vi "Copy Buffer Example.vi"() -> ()   [LabVIEW 2012]
uses:
  User Controls/Array Dimensions.ctl
  User Controls/Copy Parameters.ctl
  User Controls/Offset.ctl
  Non-User VIs/Allocate Memory/AllocateMemory_u16.vi
  Non-User VIs/Write Memory/WriteMemory_u16.vi
  Non-User VIs/Read Memory/ReadMemory 16u .vi
  Non-User VIs/Error Checking/View Error Log Mode Functional Global.vi
  OpenCLV x64.lvlib
panel:
  out "Data Out":u16[][][](array[numeric])
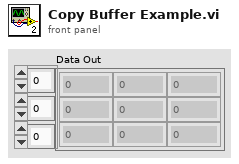
[diagram p1: front panel]
types:
  T1 = typedef "Copy Parameters.ctl" = cluster{"Source Offset":T2, "Destination Offset":T2, "Dimensions":T3}
  T2 = typedef "Offset.ctl" = cluster{"X":u64, "Y":u64, "Z":u64}
  T3 = typedef "Array Dimensions.ctl" = cluster{"Depth":u64, "Height":u64, "Width":u64}
  T4 = typedef "OpenCLV x64.lvlib/Device ID.ctl" = u64
  T5 = typedef "OpenCLV x64.lvlib/Memory Object.ctl" = cluster{"Device ID":T4, "Memeroy ID":T6, "Dimension":T3, "Memory Type":T7}
  T6 = typedef "OpenCLV x64.lvlib/Memory ID.ctl" = u64
  T7 = typedef "OpenCLV x64.lvlib/Memory Type.ctl" = enum16{"32f", "u8", "i8", "u16", "i16", "u32", "i32", "64f"}
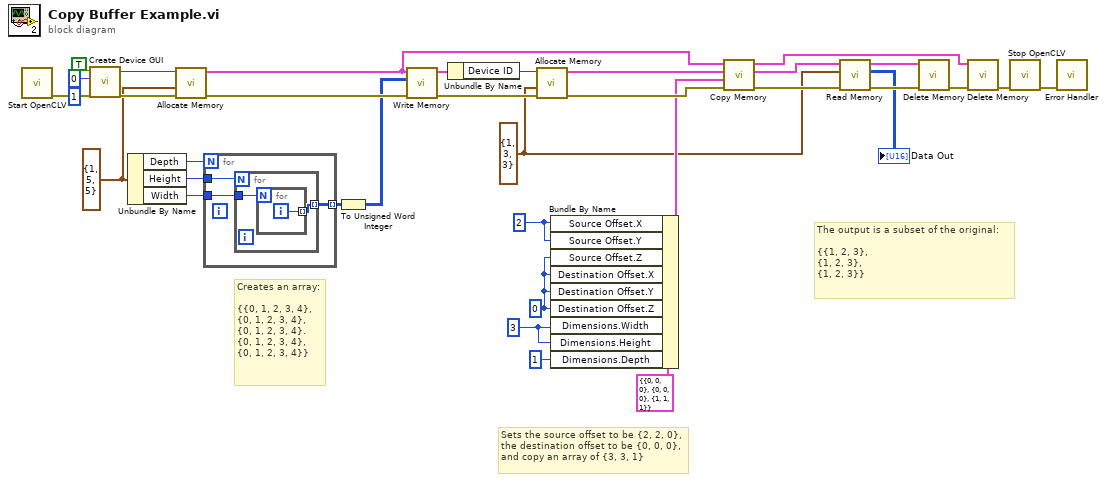
[diagram p0: block diagram]
diagram:
  w14 = u64 3 ("Dimensions.Width")
  w4 = u64 0 ("Destination Offset.Z")
  w3 = u64 2 ("Source Offset.X")
  w10 = T3 {"Depth"=1, "Height"=3, "Width"=3} ("Dimension")
  w29 = T3 {"Depth"=1, "Height"=5, "Width"=5} ("Dimension")
  # "The output is a subset of the original:\n\n{{1, 2, 3},\n{1, 2, 3},\n{1, 2, 3}}"
  # "Sets the source offset to be {2, 2, 0},\nthe destination offset to be {0, 0, 0},\nand copy an array of {3, 3, 1}"
  # "Creates an array:\n\n{{0, 1, 2, 3, 4},\n{0, 1, 2, 3, 4},\n{0, 1, 2, 3, 4}.\n{0, 1, 2, 3, 4},\n{0, 1, 2, 3, 4}}"
  n1 = call "Start OpenCLV.vi"() -> ("Error Out"=w35:errorcluster)  [unwired: 11 in]
  n2 = call "Create Device GUI.vi"("Error In"=w35, "Device"=1, "Platform"=0, "Skip Configuration"=TRUE) -> ("error constant"=w34:errorcluster, "Device Reference"=w33:T4)  [unwired: 6 in]
  n3 = Unbundle By Name(w29) -> ("Depth"=w32:u64, "Height"=w31:u64, "Width"=w26:u64)
  n4 = call-poly "Allocate Memory.vi"("Error In"=w34, "Dimension"=w29, "Device In"=w33) -> ("Error Out"=w30:errorcluster, "Memory Object"=w9:T5)  [unwired: 6 in, 1 out]
  n5 = for {
    N: w32 -> [_]
    tunnel: w31 -> [w38]
    tunnel: [w37] -> w22 mode=indexing
    tunnel: w26 -> [w36]
    n6 = for {
      N: w38 -> [_]
      tunnel: [w40] -> w37 mode=indexing
      tunnel: w36 -> [w39]
      n7 = for {
        N: w39 -> [_]
        tunnel: [w41] -> w40 mode=indexing
        i -> [w41]
      }
    }
  }
  n8 = To Unsigned Word Integer(number=w22) -> (unsigned 16bit integer=w21:u16[][][])
  n9 = call-poly "Write Memory.vi"("Error In"=w30, "Data In"=w21, "Memory Object In"=w9) -> ("Error Out"=w20:errorcluster, "Memory Object Out"=w19:T5)  [unwired: 7 in]
  n10 = Unbundle By Name(w19) -> ("Device ID"=w18:T4)
  n11 = call-poly "Allocate Memory.vi"("Error In"=w20, "Dimension"=w10, "Device In"=w18) -> ("Error Out"=w16:errorcluster, "Memory Object"=w17:T5)  [unwired: 6 in, 1 out]
  n12 = Bundle By Name(cluster=T1 {"Source Offset"={"X"=0, "Y"=0, "Z"=0}, "Destination Offset"={"X"=0, "Y"=0, "Z"=0}, "Dimensions"={"Depth"=1, "Height"=1, "Width"=1}} ("Copy Parameters"), "Source Offset.X"=w3, "Source Offset.Y"=w3, "Source Offset.Z"=w4, "Destination Offset.X"=w4, "Destination Offset.Y"=w4, "Destination Offset.Z"=w4, "Dimensions.Width"=w14, "Dimensions.Height"=w14, "Dimensions.Depth"=u64 1) -> (w12:T1)
  n13 = call "Copy Memory.vi"("Error In"=w16, "Copy Parameters"=w12, "Destination Object"=w17, "Source Object"=w9) -> ("Error Out"=w11:errorcluster, "Destination Object Out"=w2:T5, "Source Object Out"=w1:T5)  [unwired: 5 in]
  n14 = call-poly "Read Memory.vi"("Error In"=w11, "Dimensions"=w10, "Memory Object In"=w2) -> ("Error Out"=w7:errorcluster, "Data Out"=→"Data Out":u16[][][], "Memory Object Out"=w6:T5)  [unwired: 5 in, 1 out]
  n15 = call "Delete Memory.vi"("Error In"=w7, "Memory Object In"=w6) -> ("Error Out"=w8:errorcluster)  [unwired: 8 in, 1 out]
  n16 = call "Delete Memory.vi"("Error In"=w8, "Memory Object In"=w1) -> ("Error Out"=w28:errorcluster)  [unwired: 8 in, 1 out]
  n17 = call "Stop OpenCLV.vi"("Error In"=w28) -> ("Error Out"=w27:errorcluster)  [unwired: 10 in]
  n18 = call-poly "Error Handler.vi"("Error In"=w27) -> ()  [unwired: 10 in, 1 out]
